vi "Copy File Create Dirs.vi"(8 "Error In":errorcluster, 10 "Destination":path, 11 "Source":path) -> (0 "Error Out":errorcluster)   [LabVIEW 2011, in "LMH-Toolbox.lvlib" / "LMH-Common.lvlib"]
uses:
  LMH-Common.lvlib
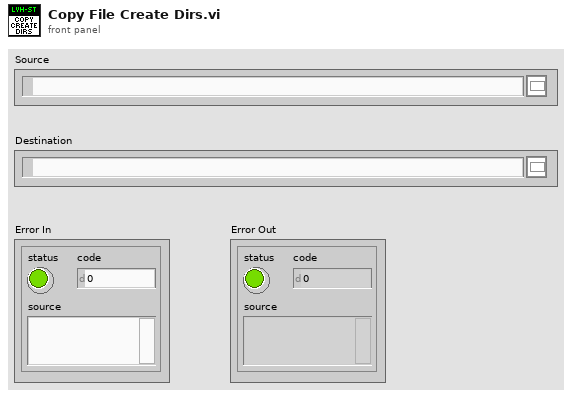
[diagram p1: front panel]
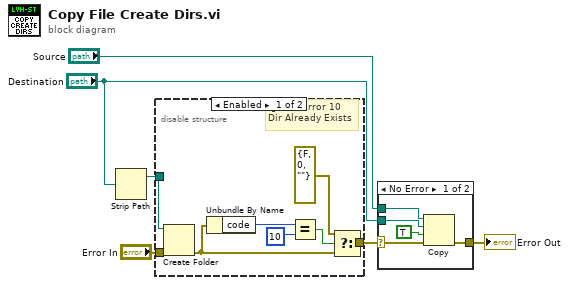
[diagram p0: block diagram]
diagram:
  n1 = Strip Path(path="Destination") -> (stripped path=w6:path)  [unwired: 1 out]
  n2 = disable-structure shown="Enabled" {
    disable-tunnel: w6 -> [w14 _]
    disable-tunnel: "Error In" -> [w13 w15]
    disable-tunnel: [w7 w15] -> w4
    frame Enabled {
      # "Ignore Error 10 \nDir Already Exists"
      n3 = Create Folder(path (use dialog)=w14, error in=w13) -> (error out=w9:errorcluster)  [unwired: 1 in, 2 out]
      n4 = Unbundle By Name(w9) -> ("code"=w12:i32)
      n5 = Equal?(x=w12, y=10) -> (x = y?=w10:bool)
      n6 = Select(t=errorcluster {"status"=FALSE, "code"=0, "source"=""}, s=w10, f=w9) -> (s? t:f=w7:errorcluster)
    }
    frame Disabled {
    }
  }
  n7 = case shown="No Error" w4 {
    selector: w4 -> [w20 w21]
    tunnel: [w19 w21] -> w3
    tunnel: "Destination" -> [w18 _]
    tunnel: "Source" -> [w17 _]
    frame No Error {
      n8 = Copy(8:w20, 9:TRUE ("overwrite (F)"), 10:w18, 11:w17) -> (0:w19:errorcluster)  [unwired: 1 in, 2 out]
    }
    frame Error {
    }
  }
  "Error Out" <- w3
